vi "合法油动机集合.vi"() -> ()   [LabVIEW 2013]
panel:
  in  "合法油动机集合":string[](array[string])=["GV", "IV", "SV", "RV", "OGV", "R2V", "I2V"]
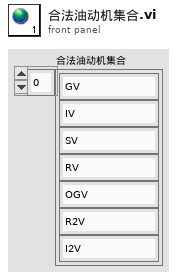
[diagram p1: front panel]
diagram:
